vi "Reserve manipulator.vi"(7 "Description":string="Reserve", 8 "Command Info":T1, 10 "Command Name":string) -> (0 "Command Info":T1)   [LabVIEW 2020]
uses:
  <vilib>/Rock Robotics/WPI/Framework/Command Status Info.ctl
  <vilib>/Rock Robotics/WPI/Framework/Completion Status.ctl
  <vilib>/Rock Robotics/WPI/Framework/Completion Notifier.ctl
  Implementation/manipulator Setpoints.ctl
  Implementation/manipulator Operations.ctl
  Implementation/Typedefs/Teleop Manipulator Commands.ctl
  Implementation/Typedefs/Cube Shooting Presets.ctl
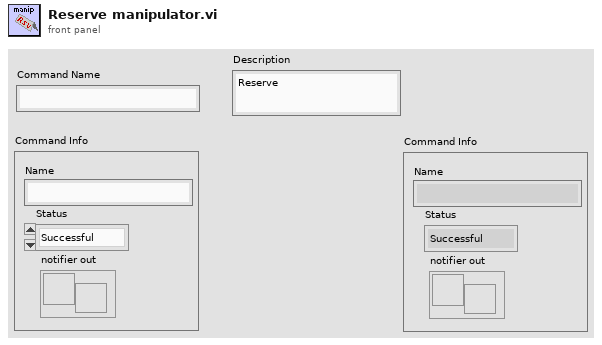
[diagram p1: front panel]
types:
  T1 = typedef "Command Status Info.ctl" = cluster{"Name":string, "Status":T2, "notifier out":T3}
  T2 = typedef "Completion Status.ctl" = enum16{"Successful", "Aborted", "Incomplete"}
  T3 = typedef "Completion Notifier.ctl" = refnum<notifier>
  T4 = typedef "manipulator Setpoints.ctl" = cluster{"Operation":T5, "Immediate Parameters":cluster{"Wrist Power":dbl, "Cascade Power":dbl}, "Griddy Parameters":cluster{"Griddy Command":T6, "Flip Wrist?":bool}, "Reset Parameters":cluster{"Reset Wrist":bool, "Reset Cascade":bool}, "Shoot Cube Parameters":cluster{"Shot Preset":T7}}
  T5 = typedef "manipulator Operations.ctl" = enum16{"Reserve", "Read Current", "Immediate", "Reset Manipulator", "Grid-dy", "Shoot Cubes"}
  T6 = typedef "Teleop Manipulator Commands.ctl" = enum16{"idle", "intake cone sideways", "intake cone upright", "intake cone feeder", "intake cube feeder", "intake cube", "score low cone", "score low cube", "score mid cone", "score mid cube", "score high cone", "score high cube", "score mid cone up"}
  T7 = typedef "Cube Shooting Presets.ctl" = enum16{"shoot low", "shoot mid", "shoot high"}
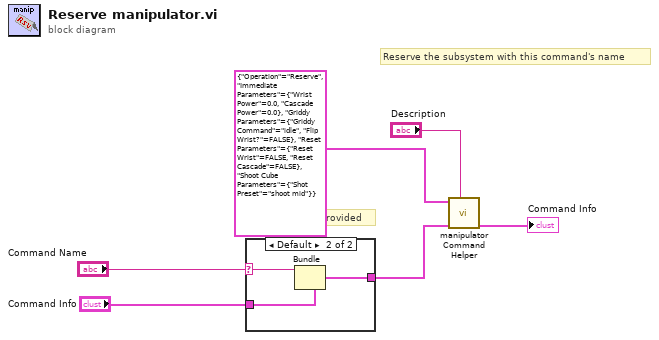
[diagram p0: block diagram]
diagram:
  # "Update name, if provided"
  # "Reserve the subsystem with this command's name"
  n1 = case shown="Default" "Command Name" {
    selector: "Command Name" -> [_ w8]
    tunnel: "Command Info" -> [w7 w10]
    tunnel: [w7 w9] -> w3
    frame "" {
    }
    frame Default {
      n2 = Bundle(cluster=w10, "Name"=w8) -> (w9:T1)  [unwired: 2 in]
    }
  }
  n3 = call "manipulator Command Helper.vi"("Description"="Description", "Command Info In"=w3, "SubSystem Data"=T4 {"Operation"=enum."Reserve", "Immediate Parameters"={"Wrist Power"=0.0, "Cascade Power"=0.0}, "Griddy Parameters"={"Griddy Command"=enum."idle", "Flip Wrist?"=FALSE}, "Reset Parameters"={"Reset Wrist"=FALSE, "Reset Cascade"=FALSE}, "Shoot Cube Parameters"={"Shot Preset"=enum."shoot mid"}}) -> ("Command Info Out"=→"Command Info":T1)  [unwired: 6 in, 2 out]
